vi "Write Raw Data Queue.vi"(8 "error in (no error)":errorcluster, 11 "Sample Buffer":u8[](array[numeric])) -> (0 "error out":errorcluster)   [LabVIEW 2016]
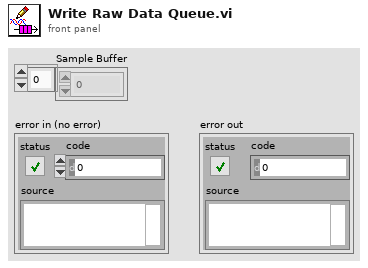
[diagram p1: front panel]
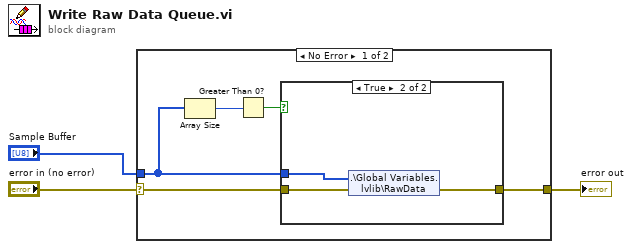
[diagram p0: block diagram]
diagram:
  n1 = case shown="No Error" "error in (no error)" {
    selector: "error in (no error)" -> [w7 w13]
    tunnel: [w8 w13] -> w3
    tunnel: "Sample Buffer" -> [w6 _]
    frame No Error {
      n2 = Array Size(array=w6) -> (size(s)=w5:i32)
      n3 = Greater Than 0?(x=w5) -> (x > 0?=w4:bool)
      n4 = case shown="True" w4 {
        tunnel: [w9 w11] -> w8
        tunnel: w7 -> [w9 w12]
        tunnel: w6 -> [_ w10]
        frame False {
        }
        frame True {
          n5 = shared-variable ".\\Global Variables.lvlib\\RawData"(w10, error in=w12) -> (error out=w11:errorcluster)
        }
      }
    }
    frame Error {
    }
  }
  "error out" <- w3
